vi "attributes-identity-test.vi"(8 "error in (no error)":errorcluster) -> (0 "error out":errorcluster)   [LabVIEW 2021]
uses:
  <vilib>/addons/_JKI Toolkits/Caraya/classes/Test/Test.lvclass
  <vilib>/addons/_JKI Toolkits/Caraya/classes/Assert/Assert.lvclass
  src/Support/Attribute.Identity/Attribute.Identity.lvclass
  src/Support/Attribute/Attribute.lvclass
  C:/Repositories/SMO/src/Support/Attribute/Attribute.lvclass
  C:/Repositories/SMO/src/Support/Attribute.Identity/Attribute.Identity.lvclass
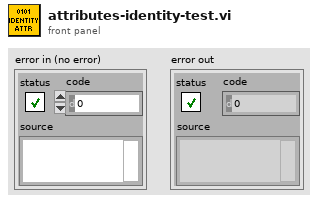
[diagram p1: front panel]
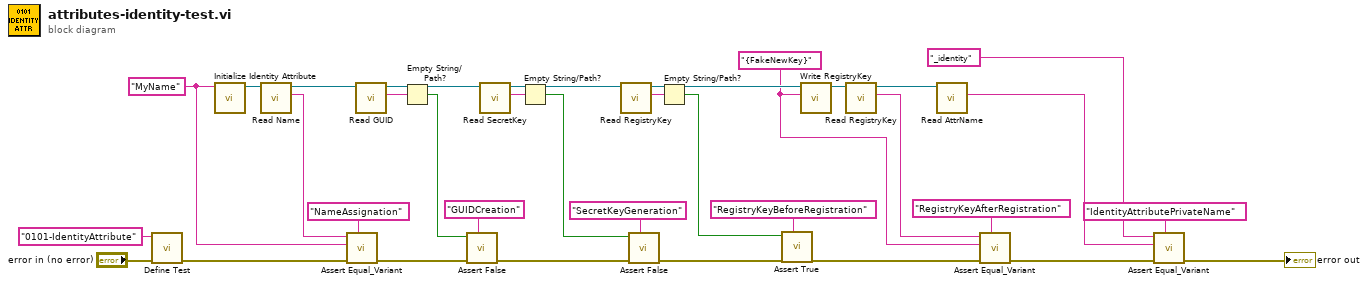
[diagram p0: block diagram]
diagram:
  w2 = "{FakeNewKey}" ("Label (VI Title)")
  w26 = "MyName" ("Name")
  n1 = call <vilib>:"Define Test.vi"("error in (no error)"="error in (no error)", "Label (VI Title)"="0101-IdentityAttribute") -> ("error out"=w33:errorcluster)  [unwired: 9 in]
  n2 = call "Initialize Identity Attribute.vi"("Given Name"=w26) -> ("Attribute.Identity"=w30:refnum<class "Attribute.Identity.lvclass">)  [unwired: 9 in, 1 out]
  n3 = call "Read Name.vi"("Attribute.Identity in"=w30) -> ("Name"=w27:string, "Attribute.Identity out"=w29:refnum<class "Attribute.Identity.lvclass">)  [unwired: 8 in, 1 out]
  n4 = call <vilib>:"Assert Equal_Variant.vi"("Label"="NameAssignation" ("Label (VI Title)"), "error in (no error)"=w33, "Y"=w26, "X"=w27) -> ("error out"=w24:errorcluster)  [unwired: 7 in]
  n5 = call "Read GUID.vi"("Attribute.Identity in"=w29) -> ("GUID"=w25:string, "Attribute.Identity out"=w28:refnum<class "Attribute.Identity.lvclass">)  [unwired: 8 in, 1 out]
  n6 = Empty String/Path?(string/path=w25) -> (empty?=w23:bool)
  n7 = call <vilib>:"Assert False.vi"("Label"="GUIDCreation" ("Label (VI Title)"), "error in (no error)"=w24, "False?"=w23) -> ("error out"=w21:errorcluster)  [unwired: 8 in]
  n8 = call "Read SecretKey.vi"("Attribute.Identity in"=w28) -> ("SecretKey"=w19:string, "Attribute.Identity out"=w17:refnum<class "Attribute.Identity.lvclass">)  [unwired: 8 in, 1 out]
  n9 = Empty String/Path?(string/path=w19) -> (empty?=w18:bool)
  n10 = call "Read RegistryKey.vi"("Attribute.Identity in"=w17) -> ("RegistryKey"=w16:string, "Attribute.Identity out"=w3:refnum<class "Attribute.Identity.lvclass">)  [unwired: 8 in, 1 out]
  n11 = call <vilib>:"Assert False.vi"("Label"="SecretKeyGeneration" ("Label (VI Title)"), "error in (no error)"=w21, "False?"=w18) -> ("error out"=w14:errorcluster)  [unwired: 8 in]
  n12 = Empty String/Path?(string/path=w16) -> (empty?=w13:bool)
  n13 = call <vilib>:"Assert True.vi"("Label"="RegistryKeyBeforeRegistration" ("Label (VI Title)"), "error in (no error)"=w14, "True?"=w13) -> ("error out"=w12:errorcluster)  [unwired: 8 in]
  n14 = call "Write RegistryKey.vi"("RegistryKey"=w2, "Attribute.Identity in"=w3) -> ("Attribute.Identity out"=w1:refnum<class "Attribute.Identity.lvclass">)  [unwired: 8 in, 1 out]
  n15 = call "Read RegistryKey.vi"("Attribute.Identity in"=w1) -> ("RegistryKey"=w11:string, "Attribute.Identity out"=w4:refnum<class "Attribute.Identity.lvclass">)  [unwired: 8 in, 1 out]
  n16 = call "Read AttrName.vi"("Attribute in"=w4) -> ("Attribute Name"=w5:string)  [unwired: 8 in, 2 out]
  n17 = call <vilib>:"Assert Equal_Variant.vi"("Label"="RegistryKeyAfterRegistration" ("Label (VI Title)"), "error in (no error)"=w12, "Y"=w2, "X"=w11) -> ("error out"=w8:errorcluster)  [unwired: 7 in]
  n18 = call <vilib>:"Assert Equal_Variant.vi"("Label"="IdentityAttributePrivateName" ("Label (VI Title)"), "error in (no error)"=w8, "Y"=w5, "X"="_identity" ("Label (VI Title)")) -> ("error out"=→"error out":errorcluster)  [unwired: 7 in]
